vi "get_json_attributes.vi"(8 "error in (no error)":errorcluster caption="entrée d'erreur (pas d'erreur)", 10 "format":string, 11 "Model en entrée":refnum<class "Model.lvclass">) -> (0 "error out":errorcluster caption="sortie d'erreur", 2 "valeur renvoyée":string, 3 "Model en sortie":refnum<class "Model.lvclass">)   [LabVIEW 2020, in "Model.lvclass"]
uses:
  Model.lvclass
  C:/Users/cipop/TDF Dropbox/2_Technologies de France/1 - Services et Etudes/PLAIY/2 - DEV/PLAIYLAB/code/Python/Python.lvclass
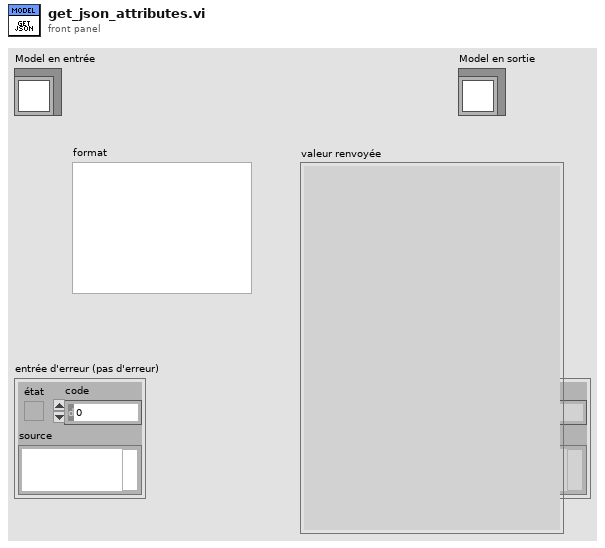
[diagram p1: front panel]
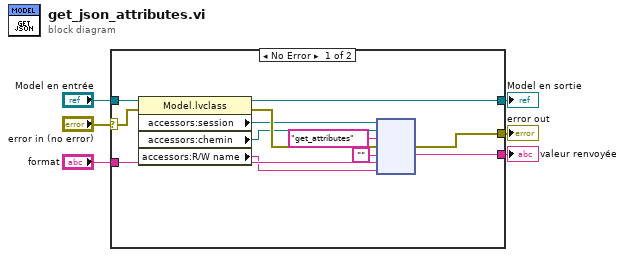
[diagram p0: block diagram]
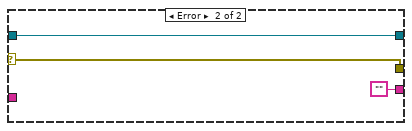
[diagram p2: hidden frame]
diagram:
  n1 = case shown="No Error" "error in (no error)" {
    selector: "error in (no error)" -> [w12 w21]
    tunnel: [w16 w21] -> w5
    tunnel: [w7 w20] -> w3
    tunnel: "Model en entrée" -> [w13 w20]
    tunnel: [w15 ""] -> w2
    tunnel: "format" -> [w14 _]
    frame No Error {
      n2 = property class="Model.lvclass"(reference=w13, error in=w12) -> (reference out=w7:refnum<class "Model.lvclass">, error out=w10:errorcluster, "accessors:session"=w9:refnum<k35>, "accessors:chemin"=w8:path, "accessors:R/W name"=w11:string)
      n3 = node(w9, w8, "get_attributes" ("nom de la fonction"), w10, "", w14, w11) -> (w16:errorcluster, w15:string)  [unwired: 2 in, 3 out]
    }
    frame Error {
    }
  }
  "error out" <- w5
  "Model en sortie" <- w3
  "valeur renvoyée" <- w2
